vi "Untitled 4.vi"() -> ()   [LabVIEW 2020]
panel:
  in  "Message 4":u64 format="%.0b"
  out "Message 3":u64 format="%.0b"
  in  "Value 2":u64 format="%.0b"
  in  "Size 2":u8
  in  "Position (0) 2":u8
  out "Position 2":u8
  out "x << y":u64
  in  "stop":bool
  out "Numeric 2":i8
  in  "Numeric":u8
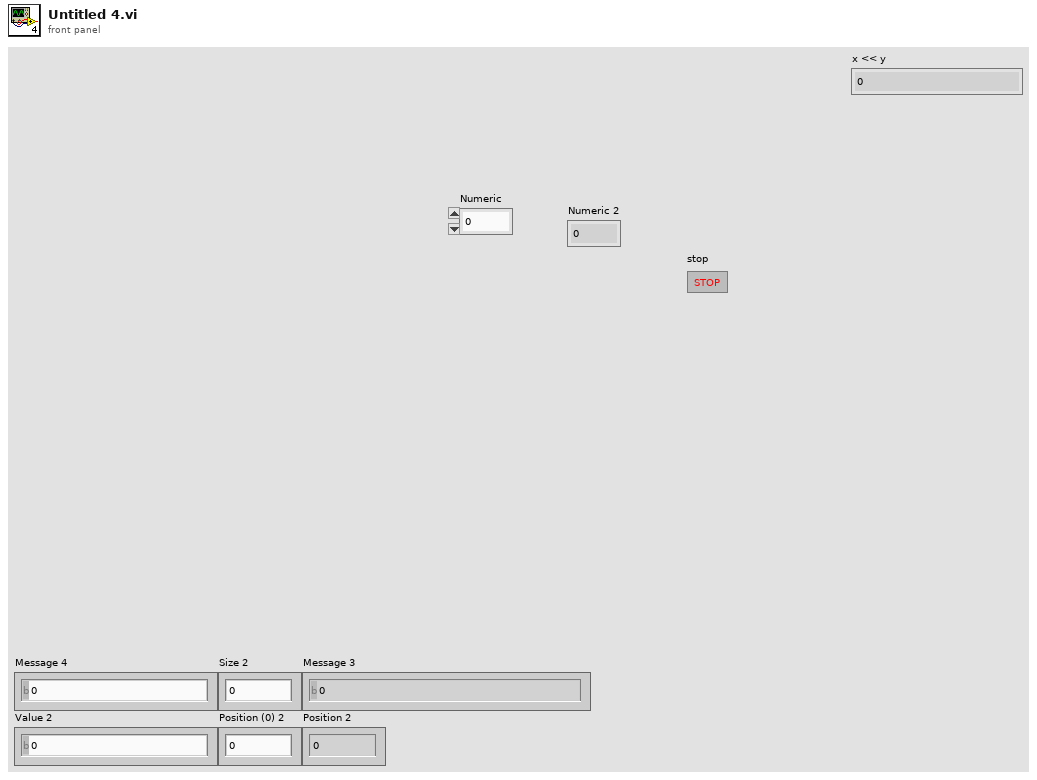
[diagram p1: front panel]
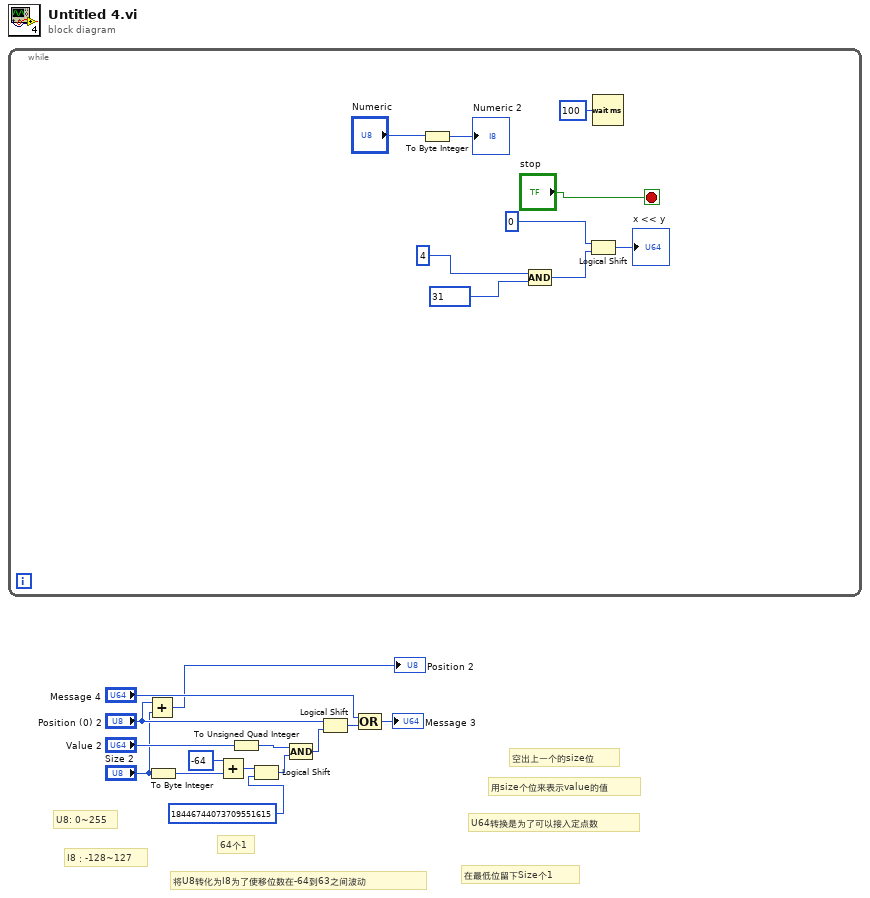
[diagram p0: block diagram]
diagram:
  # "64个1"
  # "空出上一个的size位"
  # "用size个位来表示value的值"
  # "在最低位留下Size个1"
  # "U64转换是为了可以接入定点数"
  # "将U8转化为I8为了使移位数在-64到63之间波动"
  # "I8：-128~127"
  # "U8: 0~255"
  n1 = while {
    stop <- "stop" stop-if-true
    n2 = To Byte Integer(number="Numeric") -> (8bit integer=→"Numeric 2":i8)
    n3 = Compound Arithmetic op=AND(u8 4, i64 31) -> (w18:i64)
    n4 = Logical Shift(y=0, x=w18) -> (x << y=→"x << y":i64)
    n5 = Wait (ms)(milliseconds to wait=100) -> ()  [unwired: 1 out]
  }
  n6 = Add(x="Position (0) 2", y="Size 2") -> (x+y=→"Position 2":u8)
  n7 = To Byte Integer(number="Size 2") -> (8bit integer=w1:i8)
  n8 = Add(x=i8 -64, y=w1) -> (x+y=w3:i8)
  n9 = To Unsigned Quad Integer(1:"Value 2") -> (0:w12:u64)
  n10 = Logical Shift ("逻辑移位")(y=w3, x=u64 18446744073709551615 ("value")) -> (x << y=w4:u64)
  n11 = Compound Arithmetic op=AND(w12, w4) -> (w11:u64)
  n12 = Logical Shift(y="Position (0) 2", x=w11) -> (x << y=w10:u64)
  n13 = Compound Arithmetic op=OR("Message 4", w10) -> (→"Message 3":u64)
